vi "iWorx - Pulse.vi"() -> ()   [LabVIEW 2012]
uses:
  <vilib>/measure/NI_MAPro.lvlib
  <vilib>/measure/macond.llb/IIR Filter for 1 Chan.vi
  <vilib>/DAQmx/read.llb/DAQmx Read (Analog 1D Wfm NChan NSamp).vi
  <vilib>/DAQmx/configure/timing.llb/DAQmx Timing (Sample Clock).vi
  <vilib>/DAQmx/create/channels.llb/DAQmx Create Channel (AI-Voltage-Basic).vi
panel:
  in  "Stop":bool
  in  "Reset Scale":bool
  in  "Log Info Button":bool
  out "Heart Signal":waveform(dbl)(graph)
  out "Avg Pulse":dbl format="%5.1f BPM"
  out "Inst Pulse":dbl format="%5.1f BPM"
  in  "Threshold":dbl=0.0005 step=1e-05 format="%_3pV"
  in  "Calibrate":bool
  out "error out":errorcluster
  in  "Set Up":bool
  in  "Channel":u16(ring) items=["Channel 1", "Channel 2"]
  in  "Pause Button":bool
  in  "Snapshot":bool
  in  "Clear Chart":bool
  in  "Open Log":bool
  in  "Rescale Y":bool
  out "Raw Signal":dbl(knob) scale=-0.1..0.1
  # "iWorx - Pulse - Data Logger"
  # "Sensor Input"
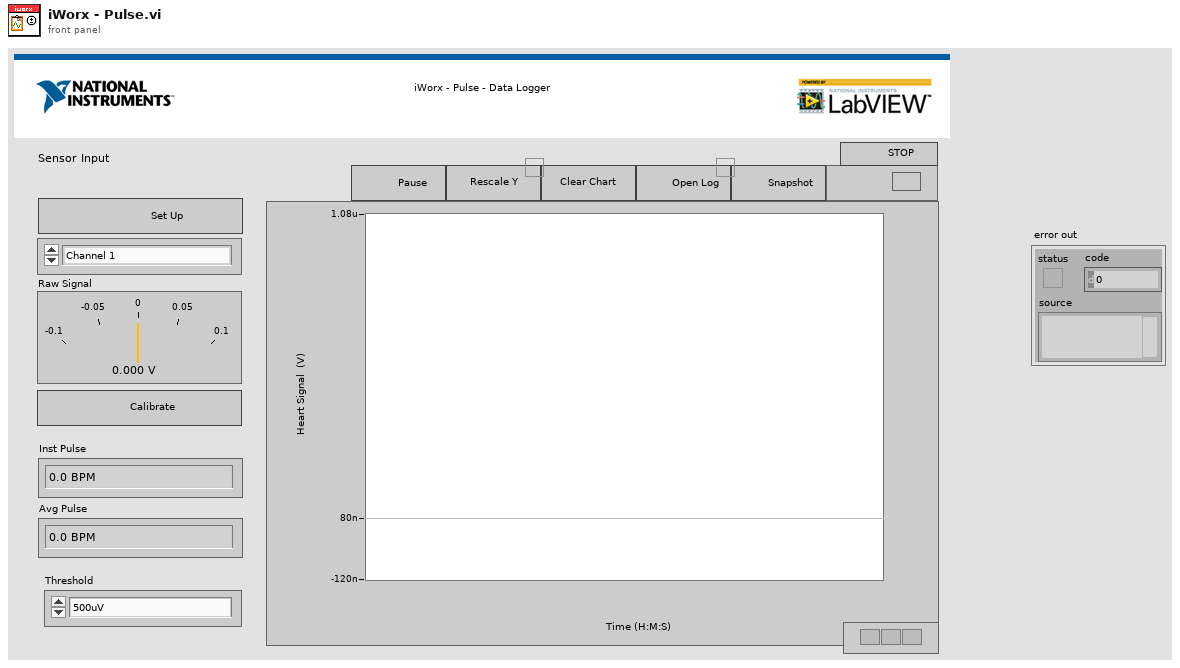
[diagram p1: front panel]
types:
  T1 = cluster{"Topology":enum16{"Off", "Butterworth", "Chebyshev", "Inverse Chebyshev", "Elliptic", "Bessel"}, "Type":enum16{"Lowpass", "Highpass", "Bandpass", "Bandstop"}, "Order":i32, "Lower Fc":dbl, "Upper Fc":dbl, "PB Ripple":dbl, "SB Attenuation":dbl}
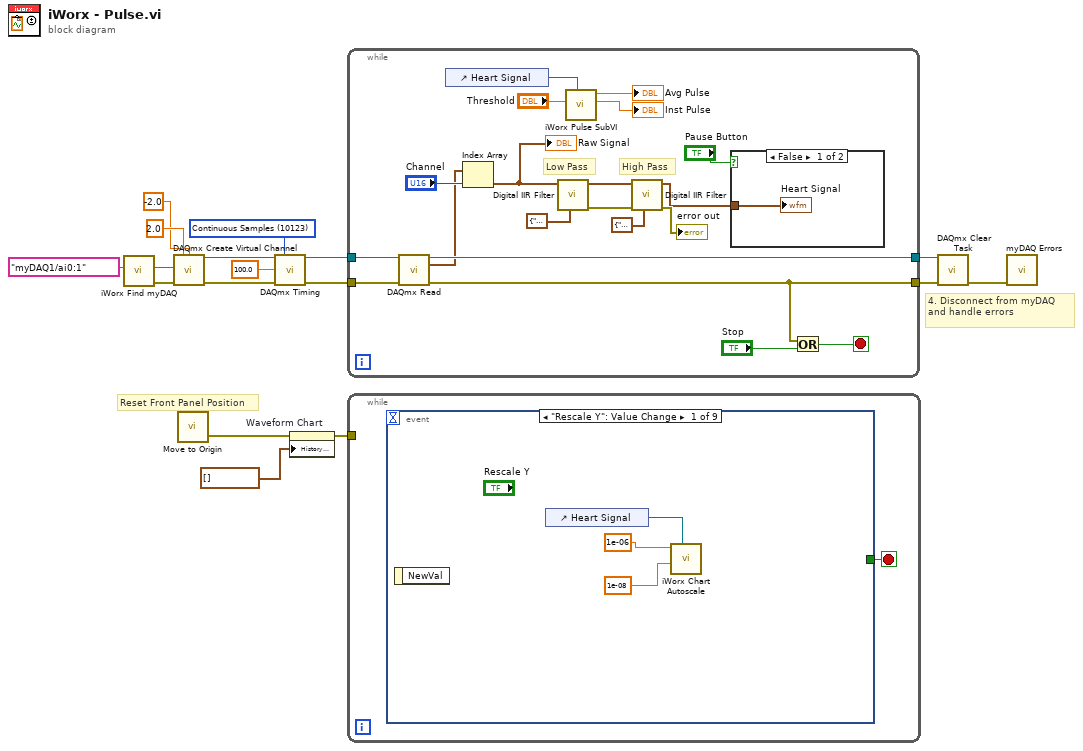
[diagram p0: block diagram]
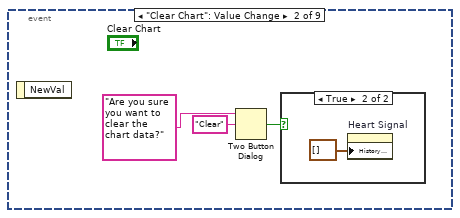
[diagram p2: hidden frame]
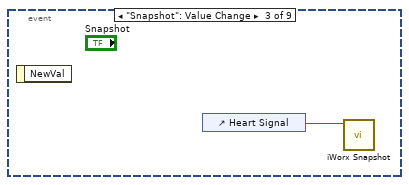
[diagram p4: hidden frame]
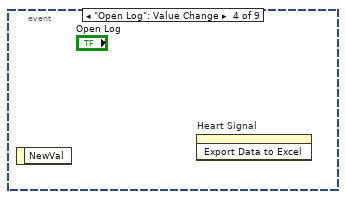
[diagram p5: hidden frame]
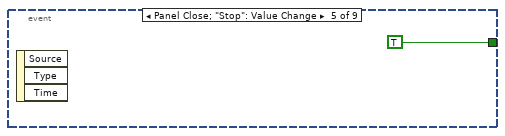
[diagram p6: hidden frame]
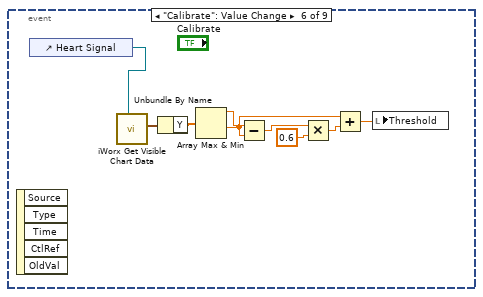
[diagram p7: hidden frame]
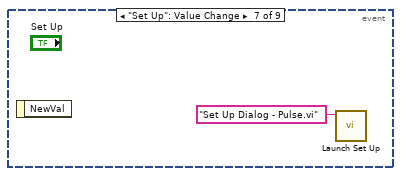
[diagram p8: hidden frame]
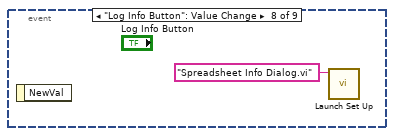
[diagram p9: hidden frame]
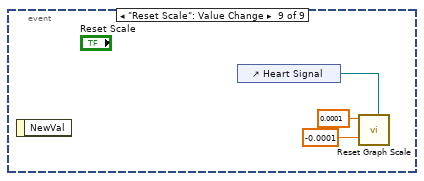
[diagram p10: hidden frame]
diagram:
  w9 = 10123 items=["Finite Samples"=10178, "Continuous Samples"=10123, "Hardware Timed Single Point"=12522] ("sample mode")
  # "4. Disconnect from myDAQ and handle errors"
  # "Reset Front Panel Position"
  n1 = call "iWorx Find myDAQ.vi"("Preferred myDAQ (myDAQ1)"=tag "myDAQ1/ai0:1" ("physical channels")) -> ("Error Out"=w5:errorcluster, "DAQmx Physical Channel"=w6:tag)  [unwired: 6 in, 3 out]
  n2 = call-poly <vilib>:"DAQmx Create Virtual Channel.vi"("maximum value"=2.0, "minimum value"=-2.0 ("maximum value"), "physical channels"=w6, "error in"=w5) -> ("task out"=w13:refnum<k21>, "error out"=w12:errorcluster)  [unwired: 10 in]
  n3 = call "Move to Origin.vi"() -> ("Error Out"=w7:errorcluster)  [unwired: 3 in]
  n4 = call-poly <vilib>:"DAQmx Timing.vi"("task/channels in"=w13, "sample mode"=w9, "rate"=100.0, "error in"=w12) -> ("task out"=w10:refnum<k21>, "error out"=w11:errorcluster)  [unwired: 10 in]
  n5 = property on="Waveform Chart" class="WFChart (strict)"(error in=w7, "History Data"=waveform(dbl)[] []) -> (error out=w14:errorcluster)  [unwired: 1 in, 1 out]
  n6 = while {
    tunnel: w10 -> [w37]
    tunnel: [w36] -> w17
    tunnel: w11 -> [w35]
    tunnel: [w33] -> w16
    stop <- w34 stop-if-true
    # "High Pass"
    # "Low Pass"
    n7 = call-poly <vilib>:"DAQmx Read.vi"("task/channels in"=w37, "error in"=w35) -> ("task out"=w36:refnum<k21>, "data"=w30:waveform(dbl)[], "error out"=w33:errorcluster)  [unwired: 11 in]
    n8 = control-ref of="Heart Signal"() -> (w23:refnum<vi>)
    n9 = Index Array(array=w30, index="Channel") -> (element=w21:waveform(dbl))
    "Raw Signal" <- w21
    n10 = call-poly <vilib>:"Digital IIR Filter.vi"("IIR filter specifications"=T1 {"Topology"=enum."Butterworth", "Type"=enum."Lowpass", "Order"=1, "Lower Fc"=0.001, "Upper Fc"=200.0, "PB Ripple"=1.0, "SB Attenuation"=60.0}, "signal in"=w21) -> ("error out"=w27:errorcluster, "signal out"=w24:waveform(dbl))  [unwired: 7 in, 1 out]
    n11 = call "iWorx Pulse SubVI.vi"("Selection Chart"=w23, "Threshold (.5mV)"="Threshold") -> ("Inst Pulse Rate (BPM)"=→"Inst Pulse":dbl, "Average Pulse Rate (BPM)"=→"Avg Pulse":dbl)  [unwired: 7 in, 1 out]
    n12 = call-poly <vilib>:"Digital IIR Filter.vi"("IIR filter specifications"=T1 {"Topology"=enum."Butterworth", "Type"=enum."Highpass", "Order"=1, "Lower Fc"=1.0, "Upper Fc"=10.0, "PB Ripple"=1.0, "SB Attenuation"=60.0} ("IIR filter specifications 2"), "error in (no error)"=w27, "signal in"=w24) -> ("error out"=→"error out":errorcluster, "signal out"=w26:waveform(dbl))  [unwired: 6 in, 1 out]
    n13 = case shown="False" "Pause Button" {
      tunnel: w26 -> [w38 _]
      frame False {
        "Heart Signal" <- w38
      }
      frame True {
      }
    }
    n14 = Or(x=w33, y="Stop") -> (x .or. y?=w34:bool)
  }
  n15 = while {
    tunnel: w14 -> [_]
    stop <- w39 stop-if-true
    n16 = event shown="[0] \"Rescale Y\": Value Change" {
      selector: _ -> [_ _ _ _ _ _ _ _ _]
      dyn-events: _ -> [_ _ _ _ _ _ _ _ _]
      timeout: _ -> [_ _ _ _ _ _ _ _ _]
      tunnel: [_ _ _ _ TRUE _ _ _ _] -> w39
      event "Rescale Y": Value Change {
        n17 = event-data() -> ()  [unwired: 1 in, 1 out]
        n18 = control-ref of="Heart Signal"() -> (w41:refnum<vi>)
        n19 = call "iWorx Chart Autoscale.vi"("Selection Chart"=w41, "Rounding Multiple (10)"=1e-08 ("Rounding Multiple (1)"), "Min Range (1)"=1e-06 ("Rounding Multiple (1)")) -> ()  [unwired: 6 in, 3 out]
      }
      event "Clear Chart": Value Change {
        n20 = event-data() -> ()  [unwired: 1 in, 1 out]
        n21 = Two Button Dialog(message="Are you sure you want to clear the chart data?", 2:"Clear" ("T button name (\"OK\")")) -> (T button?=w44:bool)  [unwired: 1 in]
        n22 = case shown="True" w44 {
          frame False {
          }
          frame True {
            n23 = property on="Heart Signal" class="WFChart (strict)"("History Data"=waveform(dbl)[] []) -> ()  [unwired: 2 in, 2 out]
          }
        }
      }
      event "Snapshot": Value Change {
        n24 = event-data() -> ()  [unwired: 1 in, 1 out]
        n25 = control-ref of="Heart Signal"() -> (w47:refnum<vi>)
        n26 = call "iWorx Snapshot.vi"("WaveformChart in"=w47) -> ()  [unwired: 10 in, 1 out]
      }
      event "Open Log": Value Change {
        n27 = event-data() -> ()  [unwired: 1 in, 1 out]
        n28 = invoke on="Heart Signal" class="WFChart (strict)" method="Export Data to Excel"() -> ()  [unwired: 3 in, 3 out]
      }
      event Panel Close; "Stop": Value Change {
        n29 = event-data() -> ()  [unwired: 1 in, 3 out]
      }
      event "Calibrate": Value Change {
        n30 = event-data() -> ()  [unwired: 1 in, 5 out]
        n31 = control-ref of="Heart Signal"() -> (w56:refnum<vi>)
        n32 = call "iWorx Get Visible Chart Data.vi"("Selection Chart"=w56) -> ("Waveform out"=w57:waveform(dbl))  [unwired: 8 in, 2 out]
        n33 = Unbundle By Name(w57) -> ("Y"=w50:dbl[])
        n34 = Array Max & Min(array=w50) -> (max value=w51:dbl, min value=w55:dbl)  [unwired: 2 out]
        n35 = Subtract(x=w51, y=w55) -> (x-y=w52:dbl)
        n36 = Multiply(x=w52, y=0.6) -> (x*y=w54:dbl)
        n37 = Add(x=w55, y=w54) -> (x+y=w49:dbl)
        n38 = local write "Threshold"(w49) -> ()
      }
      event "Set Up": Value Change {
        n39 = event-data() -> ()  [unwired: 1 in, 1 out]
        n40 = call "Launch Set Up.vi"("name or relative path"="Set Up Dialog - Pulse.vi") -> ()  [unwired: 9 in, 2 out]
      }
      event "Log Info Button": Value Change {
        n41 = event-data() -> ()  [unwired: 1 in, 1 out]
        n42 = call "Launch Set Up.vi"("name or relative path"="Spreadsheet Info Dialog.vi") -> ()  [unwired: 9 in, 2 out]
      }
      event "Reset Scale": Value Change {
        n43 = event-data() -> ()  [unwired: 1 in, 1 out]
        n44 = control-ref of="Heart Signal"() -> (w61:refnum<vi>)
        n45 = call "Reset Graph Scale.vi"("WaveformChart in"=w61, "Minimum (0)"=-0.0001, "Maximum (100)"=0.0001) -> ()  [unwired: 8 in, 1 out]
      }
    }
  }
  n46 = call <vilib>:"DAQmx Clear Task.vi"("task in"=w17, "error in"=w16) -> ("error out"=w3:errorcluster)  [unwired: 13 in]
  n47 = call "myDAQ Errors.vi"("error in (no error)"=w3) -> ()  [unwired: 10 in, 1 out]
